vi "output-cluster-data-to-file.vi"(0 "refnum in":refnum<file>, 3 "error in":errorcluster, 4 "Output - Cluster":T1 {"pHS-1" format="%.2g"; "TS-4" format="%#.2g"; "FS-2" format="%.2g"; "FS-1" format="%.2g"; "DS-1" format="%#.2g"; "DFS-1 Durchfluss" format="%#.2g"; "FS-3" format="%.2g"; "DFS-1 Volumen" format="%.0g"}) -> (7 "refnum out":refnum<file>, 10 "error out":errorcluster)   [LabVIEW 2011]
uses:
  Output - Cluster.ctl
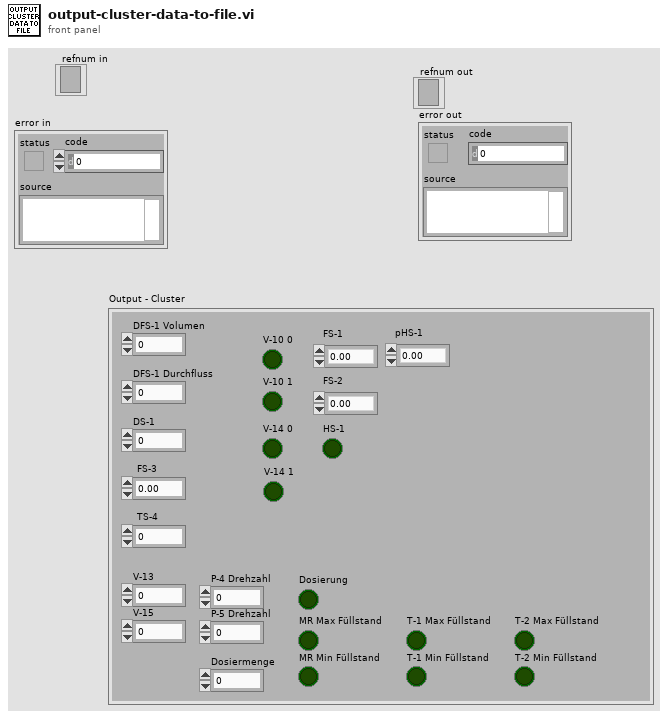
[diagram p1: front panel]
types:
  T1 = typedef "Output - Cluster.ctl" = cluster{"DFS-1 Volumen":u64, "FS-3":dbl, "DFS-1 Durchfluss":dbl, "DS-1":dbl, "V-10 0":bool, "V-14 0":bool, "FS-1":dbl, "FS-2":dbl, "TS-4":dbl, "HS-1":bool, "V-13":u8, "V-15":u8, "P-4 Drehzahl":u8, "P-5 Drehzahl":u8, "Dosierung":bool, "MR Max Füllstand":bool, "MR Min Füllstand":bool, "Dosiermenge":sgl, "V-14 1":bool, "V-10 1":bool, "T-1 Max Füllstand":bool, "T-1 Min Füllstand":bool, "T-2 Max Füllstand":bool, "T-2 Min Füllstand":bool, "pHS-1":dbl}
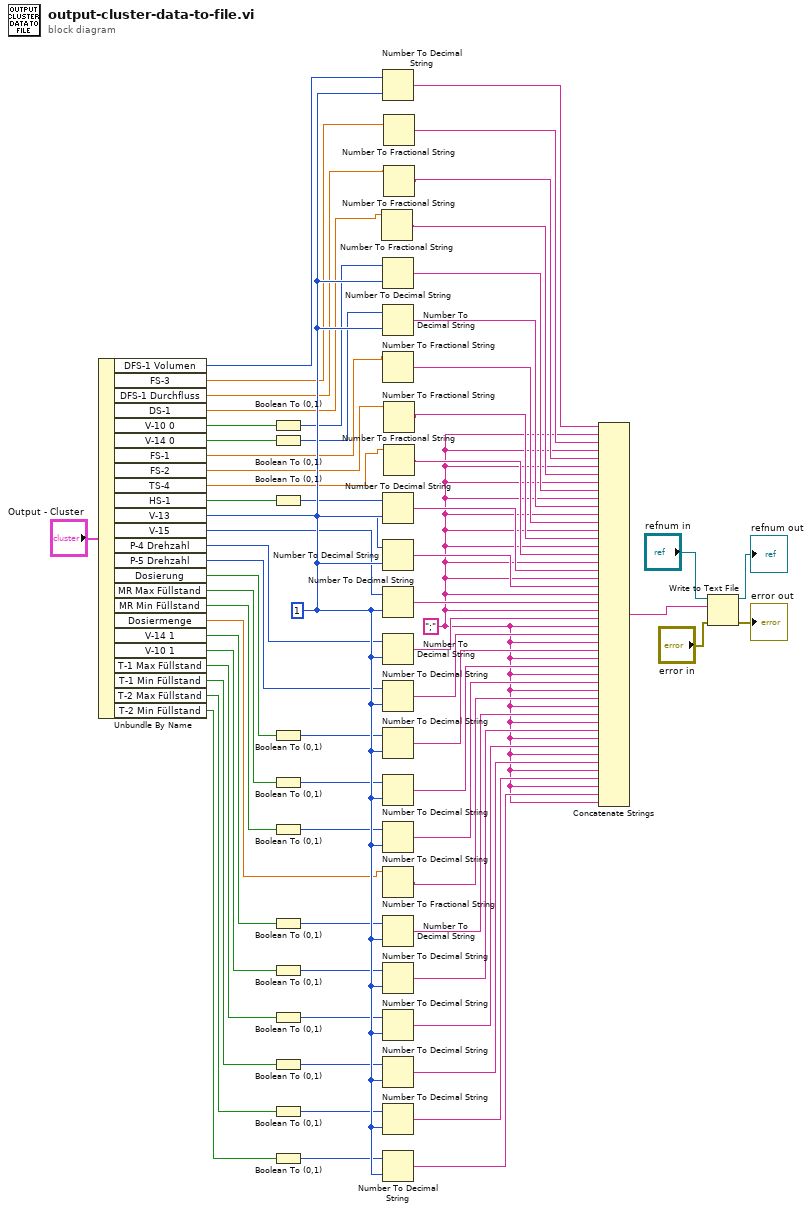
[diagram p0: block diagram]
diagram:
  w1 = ";" ("text")
  w50 = i16 1 ("width (-)")
  n1 = Unbundle By Name("Output - Cluster") -> ("DFS-1 Volumen"=w49:u64, "FS-3"=w15:dbl, "DFS-1 Durchfluss"=w12:dbl, "DS-1"=w10:dbl, "V-10 0"=w48:bool, "V-14 0"=w47:bool, "FS-1"=w6:dbl, "FS-2"=w4:dbl, "TS-4"=w3:dbl, "HS-1"=w46:bool, "V-13"=w35:u8, "V-15"=w34:u8, "P-4 Drehzahl"=w33:u8, "P-5 Drehzahl"=w32:u8, "Dosierung"=w45:bool, "MR Max Füllstand"=w44:bool, "MR Min Füllstand"=w43:bool, "Dosiermenge"=w8:sgl, "V-14 1"=w28:bool, "V-10 1"=w27:bool, "T-1 Max Füllstand"=w42:bool, "T-1 Min Füllstand"=w41:bool, "T-2 Max Füllstand"=w40:bool, "T-2 Min Füllstand"=w39:bool)
  n2 = Boolean To (0,1)(Boolean=w48) -> (0, 1=w38:i16)
  n3 = Boolean To (0,1)(Boolean=w47) -> (0, 1=w37:i16)
  n4 = Boolean To (0,1)(Boolean=w46) -> (0, 1=w36:i16)
  n5 = Boolean To (0,1)(Boolean=w45) -> (0, 1=w31:i16)
  n6 = Boolean To (0,1)(Boolean=w44) -> (0, 1=w30:i16)
  n7 = Boolean To (0,1)(Boolean=w43) -> (0, 1=w29:i16)
  n8 = Boolean To (0,1)(Boolean=w28) -> (0, 1=w26:i16)
  n9 = Boolean To (0,1)(Boolean=w27) -> (0, 1=w25:i16)
  n10 = Boolean To (0,1)(Boolean=w42) -> (0, 1=w24:i16)
  n11 = Boolean To (0,1)(Boolean=w41) -> (0, 1=w23:i16)
  n12 = Boolean To (0,1)(Boolean=w40) -> (0, 1=w22:i16)
  n13 = Boolean To (0,1)(Boolean=w39) -> (0, 1=w21:i16)
  n14 = Number To Fractional String(number=w10) -> (F-format string=w11:string)  [unwired: 3 in]
  n15 = Number To Decimal String(number=w49, width (-)=w50) -> (decimal integer string=w68:string)
  n16 = Number To Decimal String(number=w38, width (-)=w50) -> (decimal integer string=w67:string)
  n17 = Number To Decimal String(number=w37, width (-)=w50) -> (decimal integer string=w66:string)
  n18 = Number To Fractional String(number=w6) -> (F-format string=w7:string)  [unwired: 3 in]
  n19 = Number To Decimal String(number=w36, width (-)=w50) -> (decimal integer string=w65:string)
  n20 = Number To Decimal String(number=w35, width (-)=w50) -> (decimal integer string=w64:string)
  n21 = Number To Decimal String(number=w34, width (-)=w50) -> (decimal integer string=w63:string)
  n22 = Number To Decimal String(number=w33, width (-)=w50) -> (decimal integer string=w62:string)
  n23 = Number To Decimal String(number=w32, width (-)=w50) -> (decimal integer string=w61:string)
  n24 = Number To Decimal String(number=w31, width (-)=w50) -> (decimal integer string=w60:string)
  n25 = Number To Decimal String(number=w30, width (-)=w50) -> (decimal integer string=w59:string)
  n26 = Number To Decimal String(number=w29, width (-)=w50) -> (decimal integer string=w58:string)
  n27 = Number To Fractional String(number=w8) -> (F-format string=w9:string)  [unwired: 3 in]
  n28 = Number To Decimal String(number=w26, width (-)=w50) -> (decimal integer string=w57:string)
  n29 = Number To Decimal String(number=w25, width (-)=w50) -> (decimal integer string=w56:string)
  n30 = Number To Decimal String(number=w24, width (-)=w50) -> (decimal integer string=w55:string)
  n31 = Number To Decimal String(number=w23, width (-)=w50) -> (decimal integer string=w54:string)
  n32 = Number To Decimal String(number=w22, width (-)=w50) -> (decimal integer string=w53:string)
  n33 = Number To Decimal String(number=w21, width (-)=w50) -> (decimal integer string=w52:string)
  n34 = Number To Fractional String(number=w15) -> (F-format string=w14:string)  [unwired: 3 in]
  n35 = Number To Fractional String(number=w12) -> (F-format string=w13:string)  [unwired: 3 in]
  n36 = Number To Fractional String(number=w4) -> (F-format string=w5:string)  [unwired: 3 in]
  n37 = Number To Fractional String(number=w3) -> (F-format string=w2:string)  [unwired: 3 in]
  n38 = Concatenate Strings(w68, w1, w14, w1, w13, w1, w11, w1, w67, w1, w66, w1, w7, w1, w5, w1, w2, w1, w65, w1, w64, w1, w63, w1, w62, w1, w61, w1, w60, w1, w59, w1, w58, w1, w9, w1, w57, w1, w56, w1, w55, w1, w54, w1, w53, w1, w52, w1) -> (w51:string)
  n39 = Write to Text File(file (use dialog)="refnum in", text=w51, error in="error in") -> (refnum out=→"refnum out":refnum<file>, error out=→"error out":errorcluster)  [unwired: 1 in, 1 out]
